vi "Update Insert-Remove Button Enabled State.vi"(11 "UI Data in":refnum<class "Settings UI.lvclass">) -> (3 "UI Data out":refnum<class "Settings UI.lvclass">)   [LabVIEW 2020, in "Output Sequencer.lvlib" / "Settings UI.lvclass"]
uses:
  Settings UI.lvclass
  Settings UI.lvclass/Settings UI.ctl
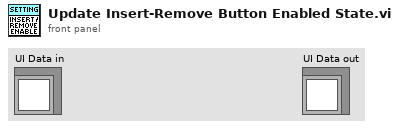
[diagram p1: front panel]
types:
  T1 = enum8{"Enabled", "Disabled", "Disabled and Grayed Out"}
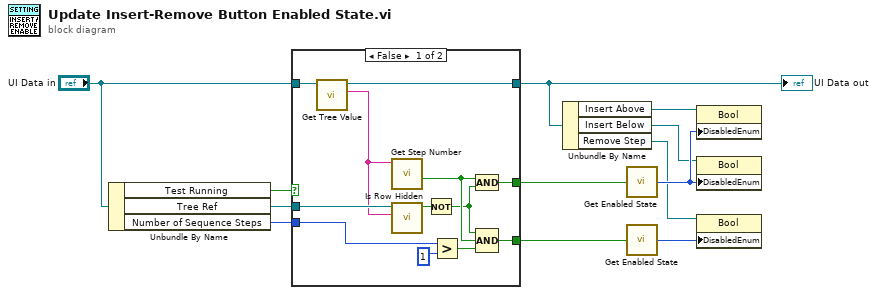
[diagram p0: block diagram]
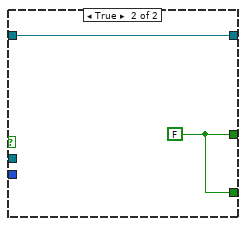
[diagram p2: hidden frame]
diagram:
  n1 = Unbundle By Name("UI Data in") -> ("Test Running"=w1:bool, "Tree Ref"=w5:refnum<vi>, "Number of Sequence Steps"=w3:i32)
  n2 = case shown="False" w1 {
    tunnel: "UI Data in" -> [w24 w25]
    tunnel: [w21 w26] -> w7
    tunnel: w5 -> [w20 _]
    tunnel: [w17 w26] -> w4
    tunnel: w3 -> [w14 _]
    tunnel: [w13 w25] -> w2
    frame False {
      n3 = call "Get Tree Value.vi"("UI Data in"=w24) -> ("Value"=w15:string, "UI Data out"=w13:refnum<class "Settings UI.lvclass">)  [unwired: 9 in]
      n4 = call "Get Step Number.vi"("Tree Tag"=w15) -> ("Is Step tag?"=w18:bool)  [unwired: 8 in, 2 out]
      n5 = call "Is Row Hidden.vi"("Tag"=w15, "TreeControl in"=w20) -> ("Hidden"=w19:bool)  [unwired: 9 in]
      n6 = Not(x=w19) -> (.not. x?=w16:bool)
      n7 = Greater?(x=w14, y=1) -> (0:w22:bool)
      n8 = Compound Arithmetic op=AND(w18, w16) -> (w17:bool)
      n9 = Compound Arithmetic op=AND(w16, w18, w22) -> (w21:bool)
    }
    frame True {
      w26 = FALSE
    }
  }
  "UI Data out" <- w2
  n10 = Unbundle By Name(w2) -> ("Insert Above"=w8:refnum<vi>, "Insert Below"=w9:refnum<vi>, "Remove Step"=w10:refnum<vi>)
  n11 = call "Get Enabled State.vi"("Enabled?"=w4) -> ("State"=w11:T1)
  n12 = call "Get Enabled State.vi"("Enabled?"=w7) -> ("State"=w6:T1)
  n13 = property on="Property Node" class="Bool"(reference=w8, "DisabledEnum"=w11) -> ()  [unwired: 1 in, 2 out]
  n14 = property on="Property Node" class="Bool"(reference=w9, "DisabledEnum"=w11) -> ()  [unwired: 1 in, 2 out]
  n15 = property on="Property Node" class="Bool"(reference=w10, "DisabledEnum"=w6) -> ()  [unwired: 1 in, 2 out]
